vi "ClassNode_Create.vi"(0 "reference":refnum<class "ClassNode.lvclass">, 5 "error in (no error)":errorcluster, 6 "GoopReferenceIn":T1) -> (14 "reference out":refnum<class "ClassNode.lvclass">, 16 "# of objects":i32, 19 "error out":errorcluster)   [LabVIEW 2012, in "ClassNode.lvclass"]
doc: "Creates and initializes a new ClassNode object.\n\nThis object should be destroyed using a ClassNode destructor VI or a virtual base class destructor VI.\n\n[GOOP 2.1]"
uses:
  <resource>/Framework/Providers/Open_GDS/UML/ClassNode_class/ClassNode.lvclass
  <resource>/Framework/Providers/Open_GDS/UML/AbstractNode_class/ObjectReference.ctl
  <resource>/Framework/Providers/Open_GDS/UML/MultiLineString_class/SizeType.ctl
  <resource>/Framework/Providers/Open_GDS/UML/MultiLineString_class/JustificationType.ctl
  <resource>/Framework/Providers/Open_GDS/UML/General/Rectangle/Rectangle Rectangle2D.ctl
  <resource>/Framework/Providers/Open_GDS/UML/RectangularNode_class/RectangularNode.lvclass
  <resource>/Framework/Providers/Open_GDS/UML/MultiLineString_class/MultiLineString.lvclass
  <resource>/Framework/Providers/Open_GDS/UML/AbstractNode_class/AbstractNode.lvclass
panel:
  # "The input reference should only\nbe wired when this method is called\nby a sub class constructor."
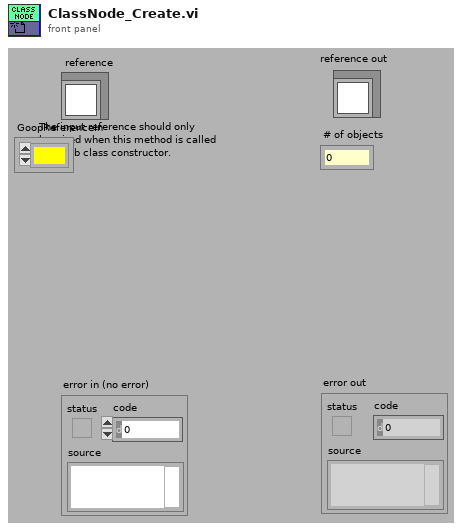
[diagram p1: front panel]
types:
  T1 = typedef "AbstractNode.lvclass/ObjectReference.ctl" = refnum<k1>
  T2 = typedef "Rectangle Rectangle2D.ctl" = cluster{"x":dbl, "y":dbl, "width":dbl, "height":dbl}
  T3 = typedef "MultiLineString.lvclass/SizeType.ctl" = enum16{"LARGE", "NORMAL", "SMALL"}
  T4 = typedef "MultiLineString.lvclass/JustificationType.ctl" = enum16{"LEFT", "CENTER", "RIGHT"}
  T5 = typedef "ClassNode.lvclass/ObjectAttributes.ctl" = cluster{"Base class":T6, "midHeight":dbl, "botHeight":dbl, "name":refnum<class "MultiLineString.lvclass">, "attributes":refnum<class "MultiLineString.lvclass">, "methods":refnum<class "MultiLineString.lvclass">, "DEFAULT_COMPARTMENT_HEIGHT":i32, "DEFAULT_WIDTH":i32, "DEFAULT_HEIGHT":i32, "showMethods":bool, "showAttributes":bool, "ClassPath":path}
  T6 = typedef "RectangularNode.lvclass/ObjectAttributes.ctl" = cluster{"Base class":T7, "bounds":T2}
  T7 = typedef "AbstractNode.lvclass/ObjectAttributes.ctl" = cluster{"parent":refnum<class "AbstractNode.lvclass">, "children":refnum<class "AbstractNode.lvclass">[], "Hidden":bool}
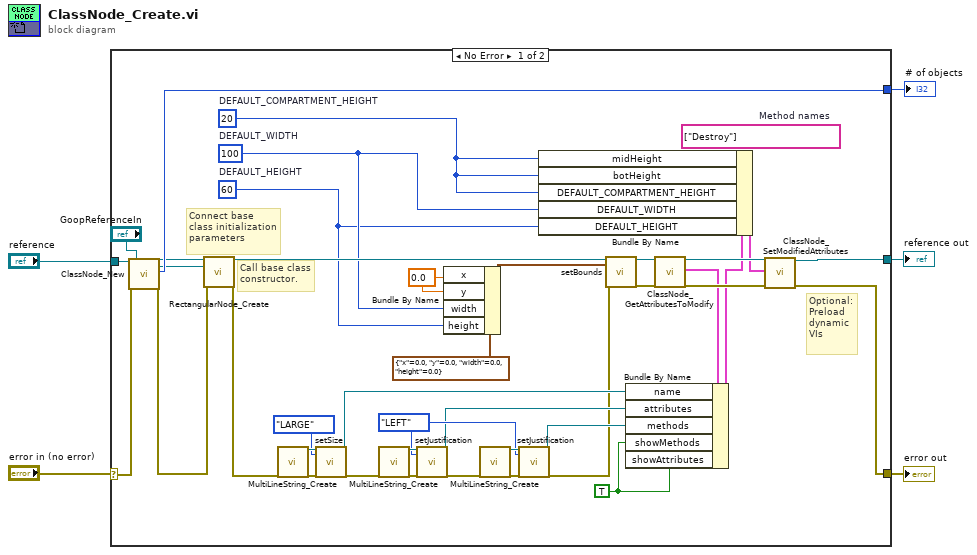
[diagram p0: block diagram]
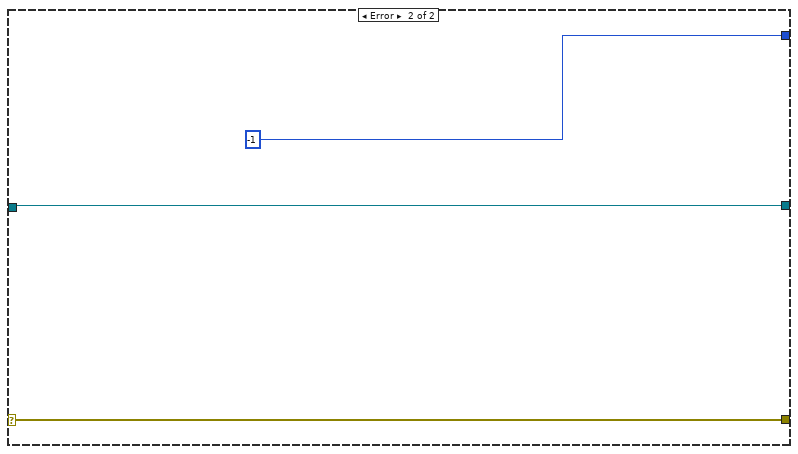
[diagram p2: hidden frame]
diagram:
  n1 = case shown="No Error" "error in (no error)" {
    selector: "error in (no error)" -> [w44 w46]
    tunnel: [w36 w45] -> w5
    tunnel: [w35 w46] -> w4
    tunnel: [w43 -1 ("Nr of open handles")] -> w3
    tunnel: "reference" -> [w42 w45]
    frame No Error {
      w14 = 0.0 ("x")
      w22 = JustificationType."LEFT" ("justification")
      (unwired) string[] ["Destroy"]  # Method names
      w9 = TRUE ("showMethods")
      w11 = 60  # DEFAULT_HEIGHT
      w13 = 100  # DEFAULT_WIDTH
      w10 = 20  # DEFAULT_COMPARTMENT_HEIGHT
      # "Optional:\nPreload\ndynamic\nVIs"
      # "Connect base\nclass initialization\nparameters"
      # "Call base class\nconstructor."
      n2 = call <resource>:"ClassNode_New.vi"("reference in"=w42, "error in (no error)"=w44, "GoopReferenceIn"="GoopReferenceIn") -> ("GoopReferenceOut"=w7:T1, "reference out"=w39:refnum<class "ClassNode.lvclass">, "# of objects"=w43:i32, "error out"=w41:errorcluster)  [unwired: 2 in, 11 out]
      n3 = call <resource>:"RectangularNode_Create.vi"("reference"=w39, "error in (no error)"=w41, "GoopReferenceIn"=w7) -> ("reference out"=w17:refnum<class "ClassNode.lvclass">, "error out"=w32:errorcluster)  [unwired: 15 out]
      n4 = call <resource>:"MultiLineString_Create.vi"("error in (no error)"=w32) -> ("reference out"=w27:refnum<class "MultiLineString.lvclass">, "error out"=w26:errorcluster)  [unwired: 3 in, 14 out]
      n5 = call <resource>:"setSize.vi"("reference"=w27, "size"=SizeType."LARGE", "error in (no error)"=w26) -> ("reference out"=w21:refnum<class "MultiLineString.lvclass">, "error out"=w25:errorcluster)  [unwired: 15 out]
      n6 = call <resource>:"MultiLineString_Create.vi"("error in (no error)"=w25) -> ("reference out"=w31:refnum<class "MultiLineString.lvclass">, "error out"=w30:errorcluster)  [unwired: 3 in, 14 out]
      n7 = call <resource>:"setJustification.vi"("reference"=w31, "justification"=w22, "error in (no error)"=w30) -> ("reference out"=w20:refnum<class "MultiLineString.lvclass">, "error out"=w24:errorcluster)  [unwired: 15 out]
      n8 = Bundle By Name(cluster=T2 {"x"=0.0, "y"=0.0, "width"=0.0, "height"=0.0} ("bounds"), "x"=w14, "y"=w14, "width"=w13, "height"=w11) -> (w16:T2)
      n9 = call <resource>:"MultiLineString_Create.vi"("error in (no error)"=w24) -> ("reference out"=w29:refnum<class "MultiLineString.lvclass">, "error out"=w28:errorcluster)  [unwired: 3 in, 14 out]
      n10 = call <resource>:"setJustification.vi"("reference"=w29, "justification"=w22, "error in (no error)"=w28) -> ("reference out"=w19:refnum<class "MultiLineString.lvclass">, "error out"=w12:errorcluster)  [unwired: 15 out]
      n11 = call-dynamic "setBounds.vi"("reference"=w17, "bounds"=w16, "error in (no error)"=w12) -> ("reference out"=w6:refnum<class "ClassNode.lvclass">, "error out"=w18:errorcluster)  [unwired: 15 in]
      n12 = call <resource>:"ClassNode_GetAttributesToModify.vi"("reference in"=w6, "error in (no error)"=w18) -> ("reference out"=w38:refnum<class "ClassNode.lvclass">, "Attributes"=w33:T5, "error out"=w40:errorcluster)  [unwired: 1 in, 14 out]
      n13 = Bundle By Name(cluster=w33, "name"=w21, "attributes"=w20, "methods"=w19, "showMethods"=w9, "showAttributes"=w9) -> (w34:T5)
      n14 = Bundle By Name(cluster=w34, "midHeight"=w10, "botHeight"=w10, "DEFAULT_COMPARTMENT_HEIGHT"=w10, "DEFAULT_WIDTH"=w13, "DEFAULT_HEIGHT"=w11) -> (w37:T5)
      n15 = call <resource>:"ClassNode_SetModifiedAttributes.vi"("reference in"=w38, "Attributes"=w37, "error in (no error)"=w40) -> ("reference out"=w36:refnum<class "ClassNode.lvclass">, "error out"=w35:errorcluster)  [unwired: 3 in, 12 out]
    }
    frame Error {
    }
  }
  "error out" <- w4
  "reference out" <- w5
  "# of objects" <- w3
